vi "set_motion_correction_parameters.vi"(6 "channel":i8, 8 "error in (no error)":errorcluster, 9 "# square points":i32, 10 "reference array":u16[][](array[numeric]), 11 "FPGAWrapperMH120124RAPS_PXI7813R in":refnum<class "FPGAWrapperMH120124RAPS_PXI7813R.lvclass">) -> (0 "error out":errorcluster, 3 "FPGAWrapperMH120124RAPS_PXI7813R out":refnum<class "FPGAWrapperMH120124RAPS_PXI7813R.lvclass">)   [LabVIEW 2010, in "FPGAWrapperMH120124RAPS_PXI7813R.lvclass"]
uses:
  FPGAWrapperMH120124RAPS_PXI7813R.lvclass
  FPGAWrapperMH120124RAPS_PXI7813R.lvclass/FPGAWrapperMH120124RAPS_PXI7813R.ctl
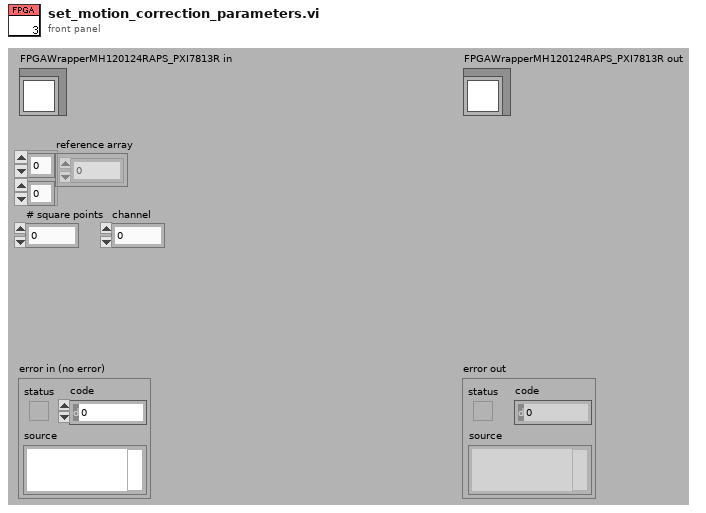
[diagram p1: front panel]
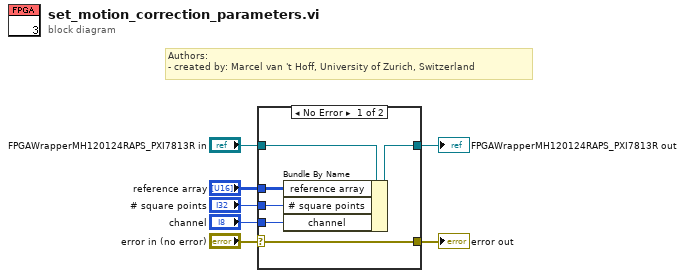
[diagram p0: block diagram]
diagram:
  # "Authors: \n- created by: Marcel van 't Hoff, University of Zurich, Switzerland"
  n1 = case shown="No Error" "error in (no error)" {
    selector: "error in (no error)" -> [w13 w15]
    tunnel: [w13 w15] -> w6
    tunnel: [w8 w14] -> w4
    tunnel: "FPGAWrapperMH120124RAPS_PXI7813R in" -> [w9 w14]
    tunnel: "reference array" -> [w12 _]
    tunnel: "# square points" -> [w11 _]
    tunnel: "channel" -> [w10 _]
    frame No Error {
      n2 = Bundle By Name(cluster=w9, "reference array"=w12, "# square points"=w11, "channel"=w10) -> (w8:refnum<class "FPGAWrapperMH120124RAPS_PXI7813R.lvclass">)
    }
    frame Error {
    }
  }
  "error out" <- w6
  "FPGAWrapperMH120124RAPS_PXI7813R out" <- w4
